vi "ADQ214 Blink (ILYA).vi"(8 "error in (no error)":errorcluster, 10 "adq214_num":i32, 11 "adq_cu_ptr in":u32) -> (0 "error out":errorcluster, 2 "return type":u32, 3 "adq_cu_ptr":u32)   [LabVIEW 2013]
uses:
  dlls/ADQAPI.dll
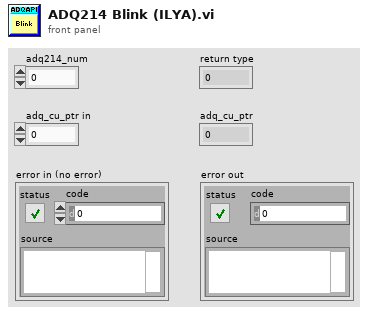
[diagram p1: front panel]
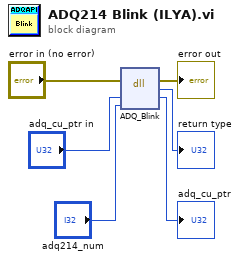
[diagram p0: block diagram]
diagram:
  n1 = dll-call lib="C:/Users/astafiev/Desktop/IlyaDrive/@photonCounting/LabView_Imperium/dlls/ADQAPI.*" fn="ADQ_Blink"(error in="error in (no error)", "adq_cu_ptr"="adq_cu_ptr in", "adq214_num"="adq214_num") -> (error out=→"error out":errorcluster, "return type"=→"return type":u32, "adq_cu_ptr"=→"adq_cu_ptr":u32)  [unwired: 3 in, 1 out]
